vi "ReferenceGen.vi"(6 "Type":string="S-shape", 7 "Num of wave":dbl=2.0 format="%#_13g", 8 "Time (s)":dbl=30.0 format="%#_13g", 9 "Amp (mm)":dbl=50.0 format="%#_13g", 10 "Sample Rate (Hz)":dbl=1000.0 format="%#_13g") -> (0 "Position Command X (mm)":dbl[](graph), 3 "Position Command Z (mm)":dbl[](graph), 5 "Freq (Hz)":dbl)   [LabVIEW 2015]
uses:
  <vilib>/Analysis/NI_AALBase.lvlib
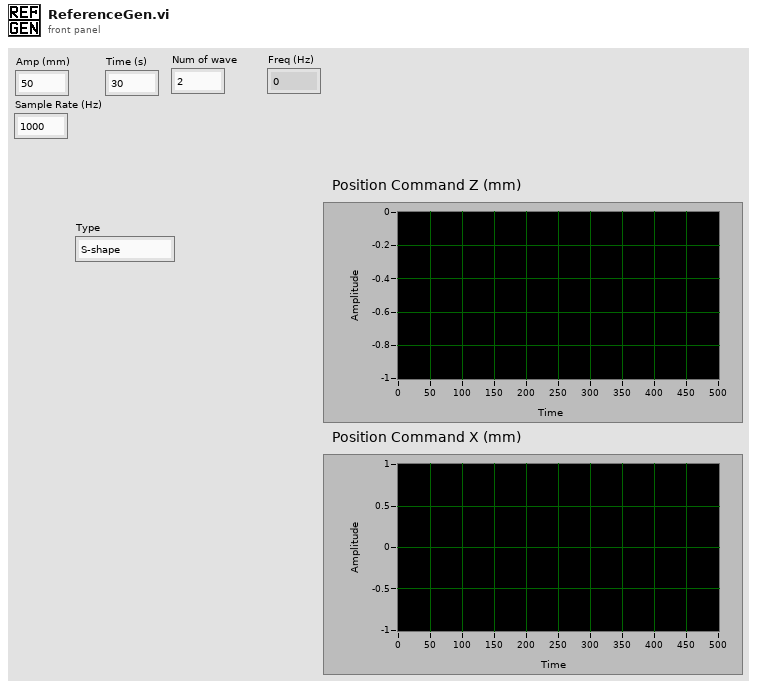
[diagram p1: front panel]
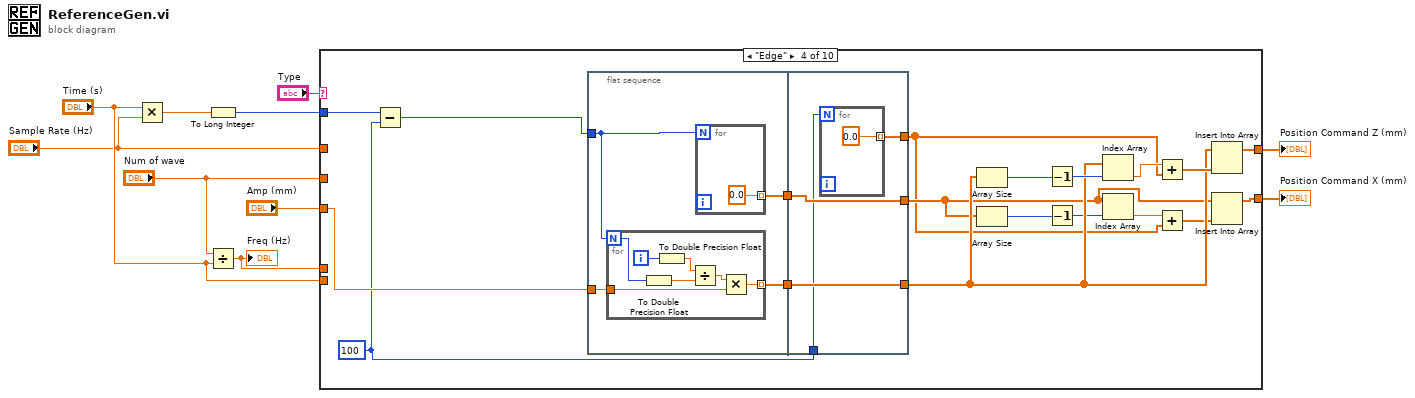
[diagram p0: block diagram]
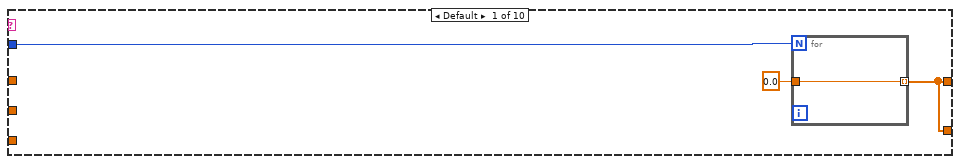
[diagram p2: hidden frame]
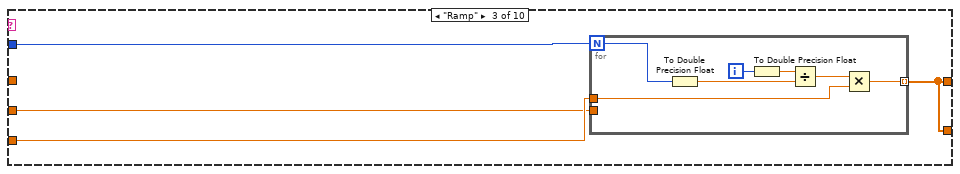
[diagram p4: hidden frame]
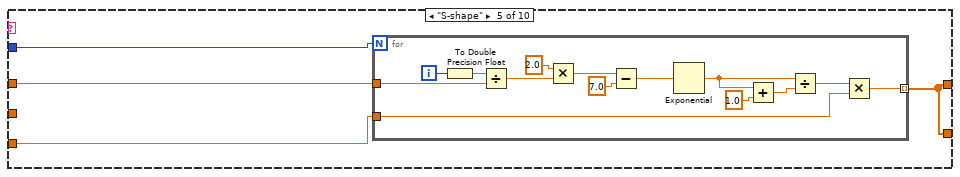
[diagram p5: hidden frame]
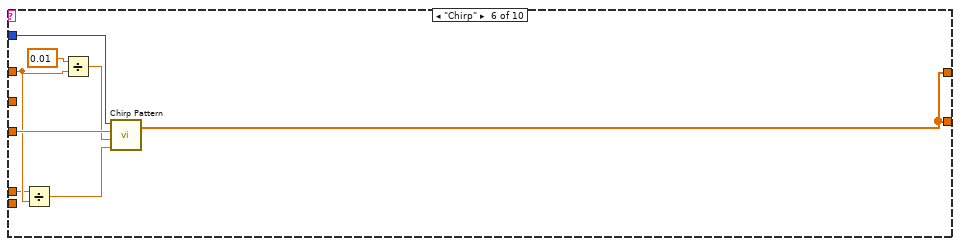
[diagram p6: hidden frame]
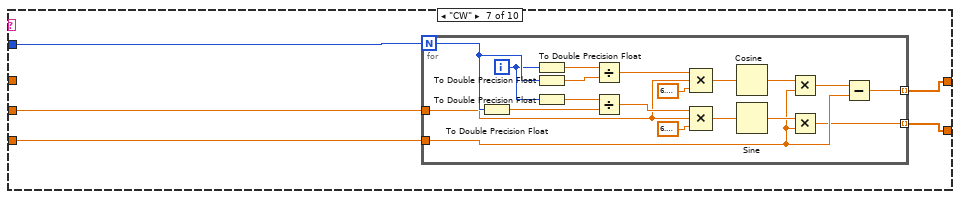
[diagram p7: hidden frame]
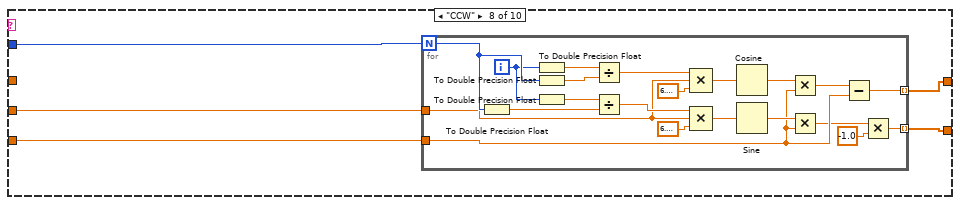
[diagram p8: hidden frame]
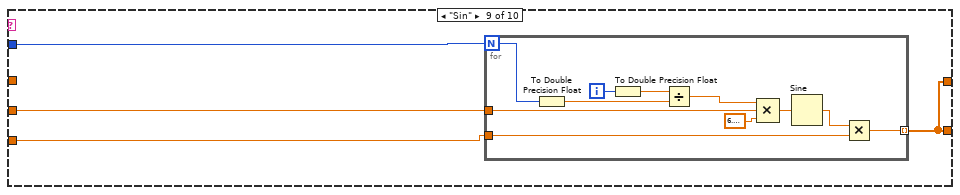
[diagram p9: hidden frame]
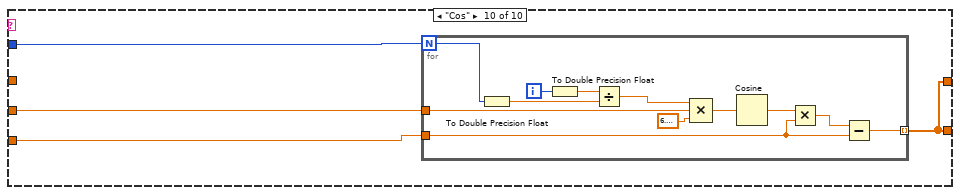
[diagram p10: hidden frame]
diagram:
  n1 = Multiply(x="Time (s)", y="Sample Rate (Hz)") -> (x*y=w8:dbl)
  n2 = To Long Integer(number=w8) -> (32bit integer=w5:i32)
  n3 = Divide(x="Num of wave", y="Time (s)") -> (x/y=w4:dbl)
  "Freq (Hz)" <- w4
  n4 = case shown="\"Edge\"" "Type" {
    tunnel: [w11 w16 w19 w38 w67 w90 w95 w117 w145 w160] -> w3
    tunnel: [w11 w16 w19 w32 w67 w90 w96 w116 w145 w160] -> w2
    tunnel: "Amp (mm)" -> [_ w17 w21 w46 w68 w91 w94 w119 w144 w159]
    tunnel: "Sample Rate (Hz)" -> [_ _ _ _ w66 w86 _ _ _ _]
    tunnel: "Num of wave" -> [_ _ w20 _ _ _ w92 w118 w142 w157]
    tunnel: "Time (s)" -> [_ _ _ _ _ _ _ _ _ _]
    tunnel: w5 -> [w13 w15 w22 w48 w69 w89 w93 w120 w143 w158]
    tunnel: w4 -> [_ _ _ _ _ w85 _ _ _ _]
    frame Default {
      n5 = for {
        N: w13 -> [_]
        tunnel: 0.0 ("Amp (mm)") -> [w14]
        tunnel: [w14] -> w11 mode=indexing
      }
    }
    frame "Const" {
      n6 = for {
        N: w15 -> [_]
        tunnel: w17 -> [w18]
        tunnel: [w18] -> w16 mode=indexing
      }
    }
    frame "Ramp" {
      n7 = for {
        N: w22 -> [w25]
        tunnel: [w27] -> w19 mode=indexing
        tunnel: w21 -> [w26]
        tunnel: w20 -> [_]
        i -> [w24]
        n8 = To Double Precision Float(number=w25) -> (double precision float=w28:dbl)
        n9 = To Double Precision Float(number=w24) -> (double precision float=w29:dbl)
        n10 = Divide(x=w29, y=w28) -> (x/y=w23:dbl)
        n11 = Multiply(x=w23, y=w26) -> (x*y=w27:dbl)
      }
    }
    frame "Edge" {
      w30 = 100 ("y")
      n12 = Subtract(x=w48, y=w30) -> (x-y=w47:i32)
      n13 = flat-sequence {
        tunnel: w47 -> [w50]
        tunnel: w46 -> [w52]
        tunnel: [w51] -> w45
        tunnel: [w49] -> w44
        tunnel: [w64] -> w39
        tunnel: w45 -> [w64]
        tunnel: w44 -> [w63]
        tunnel: [w63] -> w33
        tunnel: [w62] -> w31
        tunnel: w30 -> [w61]
        frame #0 {
          n14 = for {
            N: w50 -> [w56]
            tunnel: [w58] -> w51 mode=indexing
            tunnel: w52 -> [w57]
            i -> [w55]
            n15 = To Double Precision Float(number=w56) -> (double precision float=w59:dbl)
            n16 = To Double Precision Float(number=w55) -> (double precision float=w60:dbl)
            n17 = Divide(x=w60, y=w59) -> (x/y=w54:dbl)
            n18 = Multiply(x=w54, y=w57) -> (x*y=w58:dbl)
          }
          n19 = for {
            N: w50 -> [_]
            tunnel: [0.0] -> w49 mode=indexing
          }
        }
        frame #1 {
          n20 = for {
            N: w61 -> [_]
            tunnel: [0.0] -> w62 mode=indexing
          }
        }
      }
      n21 = Array Size(array=w39) -> (size(s)=w43:i32)
      n22 = Array Size(array=w33) -> (size(s)=w37:i32)
      n23 = Decrement(x=w43) -> (x-1=w42:i32)
      n24 = Decrement(x=w37) -> (x-1=w36:i32)
      n25 = Index Array(array=w39, index=w42) -> (element=w41:dbl)
      n26 = Index Array(array=w33, index=w36) -> (element=w35:dbl)
      n27 = Add(x=w41, y=w31) -> (x+y=w40:dbl[])
      n28 = Add(x=w35, y=w31) -> (x+y=w34:dbl[])
      n29 = Insert Into Array(array=w39, new element=w40) -> (w38:dbl[])  [unwired: 1 in]
      n30 = Insert Into Array(array=w33, new element=w34) -> (w32:dbl[])  [unwired: 1 in]
    }
    frame "S-shape" {
      n31 = for {
        N: w69 -> [_]
        tunnel: w68 -> [w70]
        tunnel: [w71] -> w67 mode=indexing
        tunnel: w66 -> [w78]
        i -> [w83]
        n32 = To Double Precision Float(number=w83) -> (double precision float=w79:dbl)
        n33 = Divide(x=w79, y=w78) -> (x/y=w77:dbl)
        n34 = Multiply(x=2.0, y=w77) -> (x*y=w75:dbl)
        n35 = Subtract(x=w75, y=7.0) -> (x-y=w74:dbl)
        n36 = Exponential(1:w74) -> (0:w81:dbl)
        n37 = Add(x=w81, y=1.0) -> (x+y=w82:dbl)
        n38 = Divide(x=w81, y=w82) -> (x/y=w72:dbl)
        n39 = Multiply(x=w72, y=w70) -> (x*y=w71:dbl)
      }
    }
    frame "Chirp" {
      n40 = Divide(x=w85, y=w86) -> (x/y=w84:dbl)
      n41 = Divide(x=0.01 ("f1"), y=w86) -> (x/y=w87:dbl)
      n42 = call <vilib>:"Chirp Pattern.vi"("f2"=w84, "f1"=w87, "amplitude"=w91, "samples"=w89) -> ("Chirp Pattern"=w90:dbl[])  [unwired: 1 out]
    }
    frame "CW" {
      n43 = for {
        N: w93 -> [w102]
        tunnel: [w97] -> w96 mode=indexing
        tunnel: [w98] -> w95 mode=indexing
        tunnel: w94 -> [w103]
        tunnel: w92 -> [w100]
        i -> [w101]
        n44 = To Double Precision Float(number=w102) -> (double precision float=w106:dbl)
        n45 = To Double Precision Float(number=w101) -> (double precision float=w113:dbl)
        n46 = To Double Precision Float(number=w102) -> (double precision float=w112:dbl)
        n47 = To Double Precision Float(number=w101) -> (double precision float=w107:dbl)
        n48 = Divide(x=w113, y=w112) -> (x/y=w111:dbl)
        n49 = Divide(x=w107, y=w106) -> (x/y=w105:dbl)
        n50 = Compound Arithmetic op=MULTIPLY(w111, w100, 6.283185307179586) -> (w115:dbl)
        n51 = Compound Arithmetic op=MULTIPLY(w105, w100, 6.283185307179586) -> (w109:dbl)
        n52 = Cosine(x=w115) -> (cos(x)=w110:dbl)
        n53 = Sine(x=w109) -> (sin(x)=w104:dbl)
        n54 = Multiply(x=w110, y=w103) -> (x*y=w99:dbl)
        n55 = Multiply(x=w104, y=w103) -> (x*y=w97:dbl)
        n56 = Subtract(x=w99, y=w103) -> (x-y=w98:dbl)
      }
    }
    frame "CCW" {
      n57 = for {
        N: w120 -> [w128]
        tunnel: [w122] -> w116 mode=indexing
        tunnel: [w124] -> w117 mode=indexing
        tunnel: w119 -> [w129]
        tunnel: w118 -> [w126]
        i -> [w127]
        n58 = To Double Precision Float(number=w128) -> (double precision float=w132:dbl)
        n59 = To Double Precision Float(number=w127) -> (double precision float=w139:dbl)
        n60 = To Double Precision Float(number=w128) -> (double precision float=w138:dbl)
        n61 = To Double Precision Float(number=w127) -> (double precision float=w133:dbl)
        n62 = Divide(x=w139, y=w138) -> (x/y=w137:dbl)
        n63 = Divide(x=w133, y=w132) -> (x/y=w131:dbl)
        n64 = Compound Arithmetic op=MULTIPLY(w137, w126, 6.283185307179586) -> (w141:dbl)
        n65 = Compound Arithmetic op=MULTIPLY(w131, w126, 6.283185307179586) -> (w135:dbl)
        n66 = Cosine(x=w141) -> (cos(x)=w136:dbl)
        n67 = Sine(x=w135) -> (sin(x)=w130:dbl)
        n68 = Multiply(x=w136, y=w129) -> (x*y=w125:dbl)
        n69 = Multiply(x=w130, y=w129) -> (x*y=w123:dbl)
        n70 = Subtract(x=w125, y=w129) -> (x-y=w124:dbl)
        n71 = Multiply(x=w123, y=-1.0) -> (x*y=w122:dbl)
      }
    }
    frame "Sin" {
      n72 = for {
        N: w143 -> [w148]
        tunnel: [w150] -> w145 mode=indexing
        tunnel: w144 -> [w149]
        tunnel: w142 -> [w146]
        i -> [w147]
        n73 = To Double Precision Float(number=w148) -> (double precision float=w153:dbl)
        n74 = To Double Precision Float(number=w147) -> (double precision float=w154:dbl)
        n75 = Divide(x=w154, y=w153) -> (x/y=w152:dbl)
        n76 = Compound Arithmetic op=MULTIPLY(w152, w146, 6.283185307179586) -> (w156:dbl)
        n77 = Sine(x=w156) -> (sin(x)=w151:dbl)
        n78 = Multiply(x=w151, y=w149) -> (x*y=w150:dbl)
      }
    }
    frame "Cos" {
      n79 = for {
        N: w158 -> [w162]
        tunnel: [w165] -> w160 mode=indexing
        tunnel: w159 -> [w164]
        tunnel: w157 -> [w161]
        i -> [w163]
        n80 = To Double Precision Float(number=w162) -> (double precision float=w169:dbl)
        n81 = To Double Precision Float(number=w163) -> (double precision float=w170:dbl)
        n82 = Divide(x=w170, y=w169) -> (x/y=w168:dbl)
        n83 = Compound Arithmetic op=MULTIPLY(w168, w161, 6.283185307179586) -> (w172:dbl)
        n84 = Cosine(x=w172) -> (cos(x)=w167:dbl)
        n85 = Multiply(x=w167, y=w164) -> (x*y=w166:dbl)
        n86 = Subtract(x=w166, y=w164) -> (x-y=w165:dbl)
      }
    }
  }
  "Position Command X (mm)" <- w2
  "Position Command Z (mm)" <- w3
